vi "Boolean Reference Read.vi"(8 "error in (no error)":errorcluster, 11 "Boolean in":refnum<vi>) -> (0 "error out":errorcluster, 3 "Value":bool)   [LabVIEW 2018]
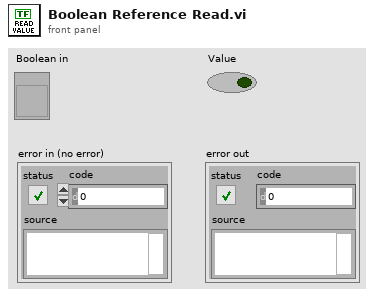
[diagram p1: front panel]
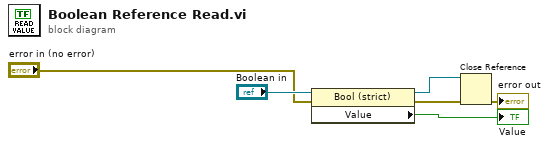
[diagram p0: block diagram]
diagram:
  n1 = property class="Bool (strict)"(reference="Boolean in", error in="error in (no error)") -> (reference out=w4:refnum<vi>, error out=w5:errorcluster, "Value"=→"Value":bool)
  n2 = Close Reference(reference=w4, error in (no error)=w5) -> (error out=→"error out":errorcluster)
